vi "get no of days in month.vi"(8 "error in (no error)":errorcluster, 10 "Year":u32, 11 "Month":T1) -> (0 "error out":errorcluster, 2 "info message":string, 3 "no. of days this month":u32)   [LabVIEW 2021, in "Project Euler.lvlib"]
uses:
  Project Euler.lvlib
  months_of_the_year enum.ctl
panel:
  # "Development\ncontrols/indicators useful for development and testing, but which are not outputs of the VI"
  # "Input\nInputs to the VI"
  # "Output\nOutputs of the VI"
  # "Description\n\nBlank VI with error handling case. \n\nSummarize the use of this VI in this space."
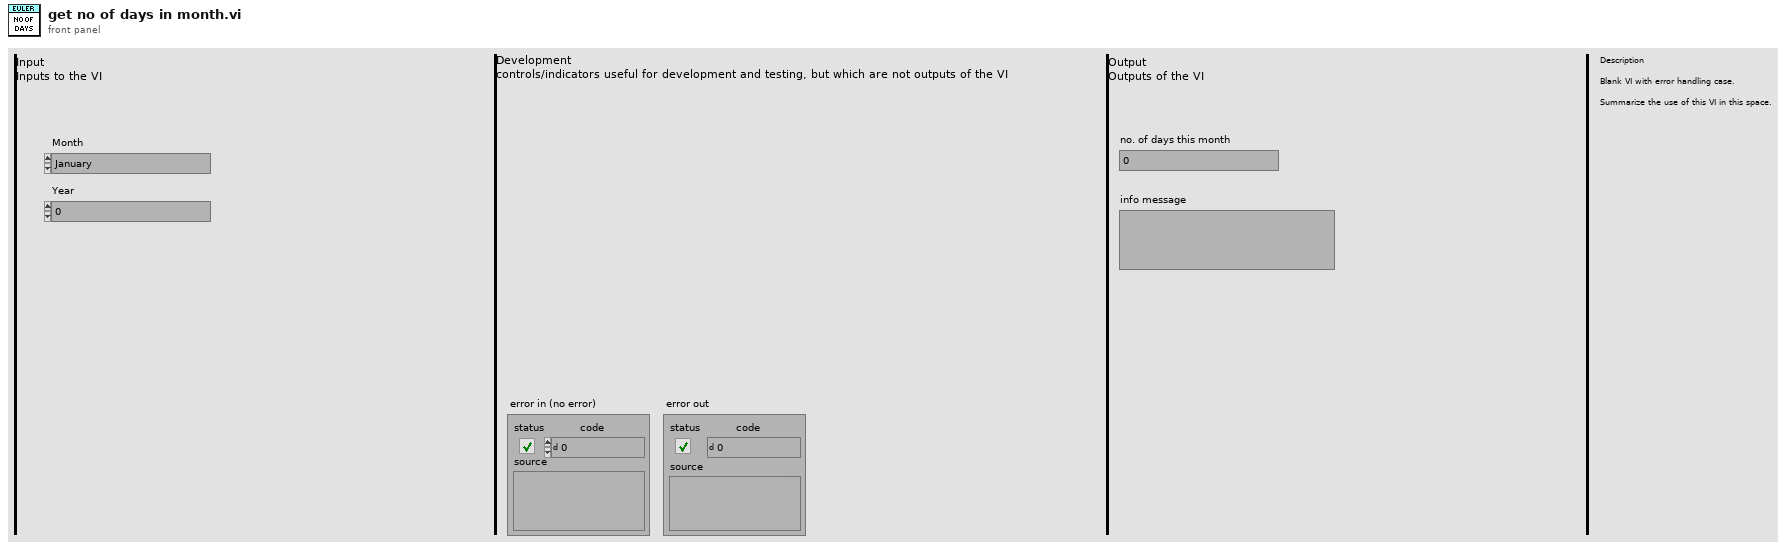
[diagram p1: front panel]
types:
  T1 = typedef "Project Euler.lvlib/months_of_the_year enum.ctl" = enum16{"January", "February", "March", "April", "May", "June", "July", "August", "September", "October", "November", "December"}
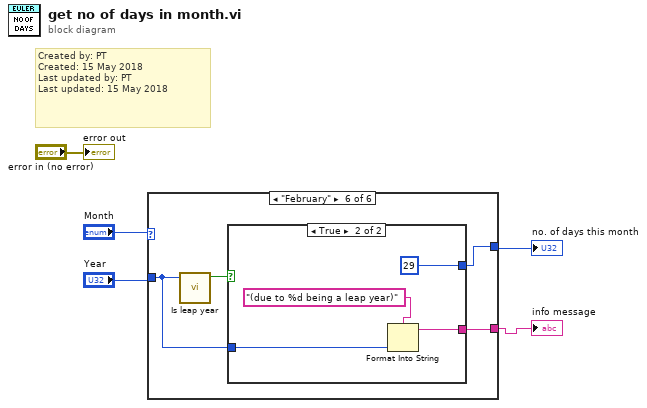
[diagram p0: block diagram]
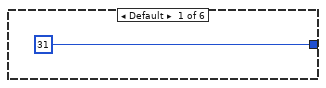
[diagram p2: hidden frame]
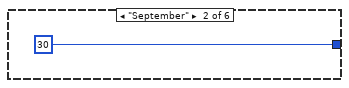
[diagram p3: hidden frame]
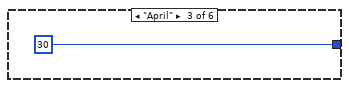
[diagram p4: hidden frame]
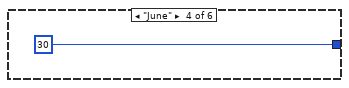
[diagram p5: hidden frame]
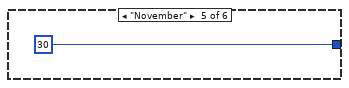
[diagram p6: hidden frame]
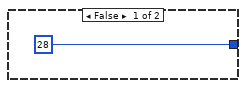
[diagram p7: hidden frame]
diagram:
  # "Created by: PT\nCreated: 15 May 2018\nLast updated by: PT\nLast updated: 15 May 2018"
  n1 = case shown="\"February\"" "Month" {
    tunnel: [u32 31 ("lower limit") u32 30 ("lower limit") u32 30 ("lower limit") u32 30 ("lower limit") u32 30 ("lower limit") w14] -> w1
    tunnel: "Year" -> [_ _ _ _ _ w12]
    tunnel: [_ _ _ _ _ w11] -> w2
    frame Default {
    }
    frame "September" {
    }
    frame "April" {
    }
    frame "June" {
    }
    frame "November" {
    }
    frame "February" {
      n2 = call "Is leap year.vi"("Year"=w12) -> ("T = input is leap year"=w13:bool)  [unwired: 8 in, 2 out]
      n3 = case shown="True" w13 {
        tunnel: [u32 28 ("lower limit") u32 29 ("lower limit")] -> w14
        tunnel: w12 -> [_ w17]
        tunnel: [_ w16] -> w11
        frame False {
        }
        frame True {
          n4 = Format Into String(format string="(due to %d being a leap year)", w17) -> (resulting string=w16:string)  [unwired: 2 in, 1 out]
        }
      }
    }
  }
  "no. of days this month" <- w1
  "info message" <- w2
  "error out" <- "error in (no error)"
